vi "fgt get pressure channels Info.vi"(8 "error in (no error)":errorcluster) -> (0 "error out":errorcluster, 3 "Pressure channels info":T1[](array[typedef]) {"indexID" format="%.0x"; "index" format="%.0x"; "position" format="%.0x"; "DeviceSN" format="%.0x"; "firmware" format="%.0x"; "ControllerSN" format="%.0x"})   [LabVIEW 2016, in "fgt_SDK.lvlib"]
doc: "Get total number of initialized pressure channels. It is the sum of all MFCS, MFCS-EZ and FlowEZ pressure controllers"
uses:
  fgt_SDK.lvlib
  TypeDefs/fgt_CHANNEL_INFO.ctl
  TypeDefs/fgt_INSTRUMENT_TYPE.ctl
  dlls/fgt_SDK_32.dll
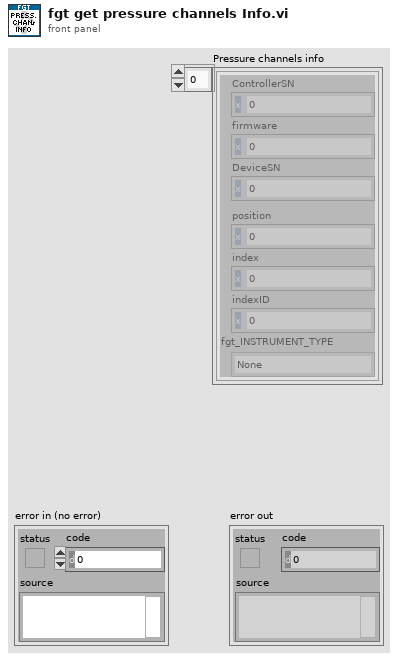
[diagram p1: front panel]
types:
  T1 = typedef "fgt_SDK.lvlib/fgt_CHANNEL_INFO.ctl" = cluster{"ControllerSN":u16, "firmware":u16, "DeviceSN":u16, "position":u32, "index":u32, "indexID":u32, "fgt_INSTRUMENT_TYPE":T2}
  T2 = typedef "fgt_SDK.lvlib/fgt_INSTRUMENT_TYPE.ctl" = enum32{"None", "MFCS", "MFCS_EZ", "FRP", "LineUP"}
  T3 = cluster{"ControllerSN":u16, "firmware":u16, "DeviceSN":u16, "Padding":u16, "position":u32, "index":u32, "indexID":u32, "fgt_INSTRUMENT_TYPE":T2}
  T4 = cluster{"ControllerSN":u16, "firmware":u16, "DeviceSN":u16, "Padding":u16, "position":u32, "index":u32, "indexID":u32, "fgt_INSTRUMENT_TYPE":T2}[]
  T5 = typedef "fgt_SDK.lvlib/fgt_STATUS_INFO.ctl" = cluster{"InstrType":T2, "instrSN":u16, "errorCode":u8, "infoCode":u8, "detail":string}
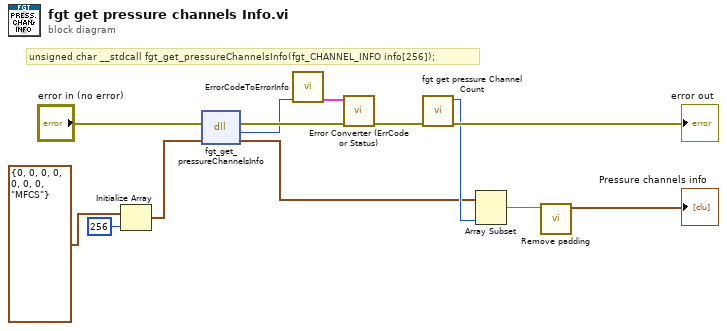
[diagram p0: block diagram]
diagram:
  # "unsigned char __stdcall fgt_get_pressureChannelsInfo(fgt_CHANNEL_INFO info[256]);"
  n1 = Initialize Array(T3 {"ControllerSN"=0, "firmware"=0, "DeviceSN"=0, "Padding"=0, "position"=0, "index"=0, "indexID"=0, "fgt_INSTRUMENT_TYPE"=enum."MFCS"} ("fgt_CHANNEL_INFO"), 256 ("dimension size")) -> (w7:T4)
  n2 = dll-call lib="PTH2Zabs D\nMes DocumentsDéveloppementFluigentSDKsfgt-sdk-labviewdllsfgt_SDK_*.*" fn="fgt_get_pressureChannelsInfo"(error in="error in (no error)", "info"=w7) -> (error out=w12:errorcluster, "return type"=w11:u8, "info"=w3:T4)  [unwired: 2 in, 1 out]
  n3 = call "ErrorCodeToErrorInfo.vi"("return type"=w11) -> ("StatusInfo"=w10:T5)  [unwired: 10 in]
  n4 = call "Error Converter (ErrCode or Status).vi"("error in (no error)"=w12, "StatusInfo"=w10) -> ("error out"=w6:errorcluster)  [unwired: 9 in]
  n5 = call "fgt get pressure Channel Count.vi"("error in (no error)"=w6) -> ("error out"=→"error out":errorcluster, "nbPChan out"=w4:u32)  [unwired: 9 in]
  n6 = Array Subset(array=w3, length=w4) -> (w1:T4)  [unwired: 1 in]
  n7 = call "Remove padding.vi"("Array in"=w1) -> ("Array out"=→"Pressure channels info":T1[])  [unwired: 10 in]
